vi "EnqueueDrive.vi"(0 "cDriveLeft":dbl, 1 "LoopTiming":u32, 5 "cDriveRight":dbl, 7 "cHalfDrive":bool, 9 "cStraightDrive":bool, 11 "error in (no error)":errorcluster) -> (15 "error out":errorcluster)   [LabVIEW 2013]
uses:
  DriveQueueInstruction.ctl
  DriveInstruction.ctl
  QueueSubsystem.ctl
  DriveAction.ctl
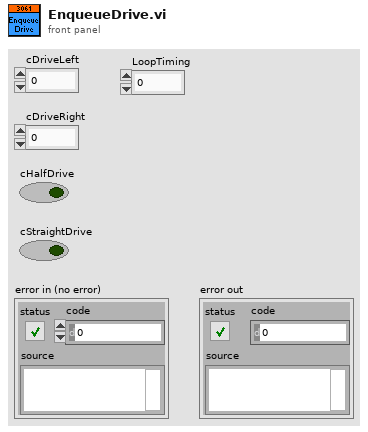
[diagram p1: front panel]
types:
  T1 = typedef "DriveAction.ctl" = enum16{"Init", "LinearDrive", "SetValue", "Disable"}
  T2 = typedef "QueueSubsystem.ctl" = enum16{"Drive", "Arm", "Catapult", "Roller"}
  T3 = typedef "DriveQueueInstruction.ctl" = cluster{"DriveInstruction":T4, "Subsystem":T2, "DriveAction":T1, "LoopTiming":u32}
  T4 = typedef "DriveInstruction.ctl" = cluster{"cDriveLeft":dbl, "cDriveRight":dbl, "cHalfDrive":bool, "cStraightDrive":bool}
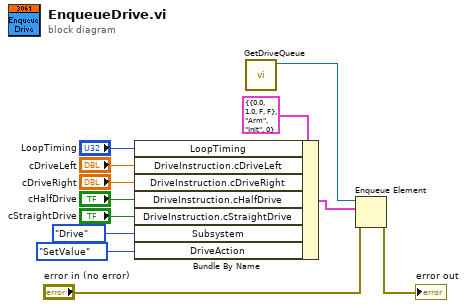
[diagram p0: block diagram]
diagram:
  n1 = Bundle By Name(cluster=T3 {"DriveInstruction"={"cDriveLeft"=0.0, "cDriveRight"=1.0, "cHalfDrive"=FALSE, "cStraightDrive"=FALSE}, "Subsystem"=enum."Arm", "DriveAction"=enum."Init", "LoopTiming"=0} ("DriveQueueInstruction"), "LoopTiming"="LoopTiming", "DriveInstruction.cDriveLeft"="cDriveLeft", "DriveInstruction.cDriveRight"="cDriveRight", "DriveInstruction.cHalfDrive"="cHalfDrive", "DriveInstruction.cStraightDrive"="cStraightDrive", "Subsystem"=QueueSubsystem."Drive", "DriveAction"=DriveAction."SetValue") -> (w3:T3)
  n2 = call "GetDriveQueue.vi"() -> ("queue out"=w6:refnum<queue>)  [unwired: 10 in, 1 out]
  n3 = Enqueue Element(queue=w6, element=w3, error in (no error)="error in (no error)") -> (error out=→"error out":errorcluster)  [unwired: 1 in, 2 out]
